vi "Create Installer.vi"(0 "Project Refnum":refnum<vi>, 5 "Build specification name":string, 11 "error in (no error)":errorcluster) -> (4 "Project Refnum Out":refnum<vi>, 15 "error out":errorcluster)   [LabVIEW 2021, in "G-Plugin Editor.lvlib"]
uses:
  G-Plugin Editor.lvlib
  <vilib>/AppBuilder/IB_Classes/Installer/Installer.lvclass
  <vilib>/AppBuilder/AB_API/common/AB_API Build Object Type.ctl
  <vilib>/AppBuilder/IB_Classes/Source/IB_Source.ctl
  <vilib>/AppBuilder/IB_Classes/Source/Container/Build/PackedLib/IB_PackedLib.lvclass
  C:/Program Files/National Instruments/LabVIEW 2021/vi.lib/AppBuilder/IB_Classes/Source/IB_Source.lvclass
  <vilib>/AppBuilder/IB_Classes/Destination/absFolder/absFolder.lvclass
  C:/Program Files/National Instruments/LabVIEW 2021/vi.lib/AppBuilder/IB_Classes/Destination/IB_Destination.lvclass
  <vilib>/AppBuilder/IB_Classes/Source/IB_Source.lvclass
  <vilib>/AppBuilder/IB_Classes/Destination/IB_Destination.lvclass
panel:
  out "Class out":refnum<class "Installer.lvclass">
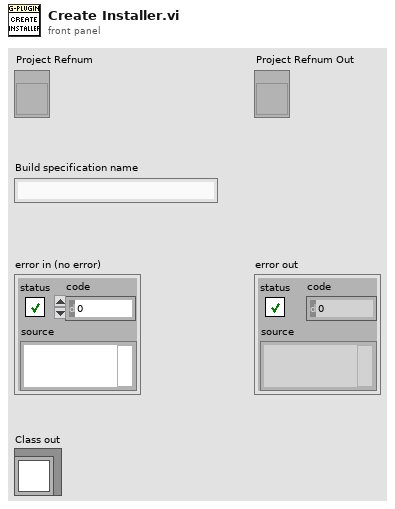
[diagram p1: front panel]
types:
  T1 = typedef "IB_Source.ctl" = cluster{"name":string, "sourceTag":string, "destTag":string, "path":path, "eng_installPath":string, "UI_inBuild?":bool, "str ref?":bool}
  T2 = typedef "AB_API Build Object Type.ctl" = enum16{"Source Distribution", "DLL", "EXE", "Installer", "Zip File", "RESTful WS", "RTEXE", "Packed Library", "C Generation ", ".NET Interop Assembly"}
  T3 = typedef "ItemRef.ctl" = u64
  T4 = typedef "IB_Installer.ctl" = cluster{"Destination":refnum<class "IB_Destination.lvclass">[], "Source":refnum<class "IB_Source.lvclass">[], "buildObject":T3, "defaultDir":string, "platform":string, "author":string, "productName":string, "buildSpecName":string, "hide":bool, "requireLVDevSys":bool, "autoIncrement":bool, "includeError":bool, "readmeID":string, "buildLocation":path, "readmePath":path, "mediaSize":u16, "language":T5, "productVersion":T6, "preview":bool, "programmatic":bool, "progressBarEvents":T7, "userLog_Path":path, "shortcutAddresses":T9[], "EXE_Install Address":string, "EXE_Uninstall Address":string, "additional NIPaths":refnum<class "Dest_NI_NIPath.lvclass">[], "web service itemIDs":string[], "installerName":string}
  T5 = typedef "CDK_sTypeDef_Languages.ctl" = u16
  T6 = typedef "CDK_sTypeDef_ProductVersion.ctl" = cluster{"Major":u8, "Minor":u8, "Update":u16}
  T7 = typedef "provcom_ProgressBar_Events.ctl" = cluster{"newJob":refnum<user-event>, "newItem":refnum<user-event>, "errorMsg":T8, "cancel":refnum<user-event>}
  T8 = typedef "mxLvBuildError.ctl" = refnum<user-event>
  T9 = typedef "CDK_sTypeDef_ShortcutAddress.ctl" = cluster{"file":string, "shortcut":string}
  T10 = typedef "IB_Destination.ctl" = cluster{"name":string, "unlock":bool, "parentTag":string, "destTag":string, "eng_installPath":string}
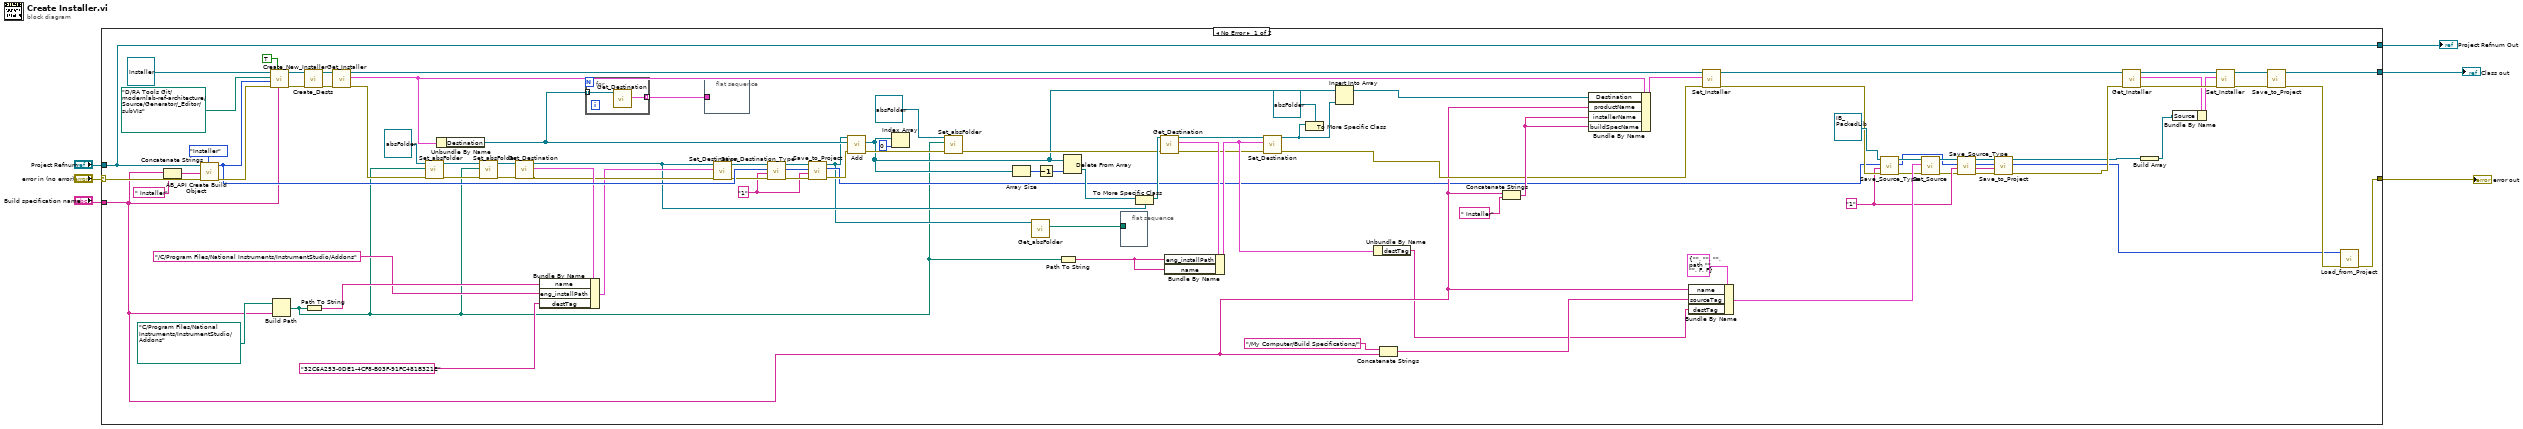
[diagram p0: block diagram]
diagram:
  n1 = case shown="No Error" "error in (no error)" {
    selector: "error in (no error)" -> [w100 w105]
    tunnel: [w72 w105] -> w6
    tunnel: "Build specification name" -> [w34 _]
    tunnel: "Project Refnum" -> [w91 w104]
    tunnel: [w88 _] -> w2
    tunnel: [w91 w104] -> w1
    frame No Error {
      w28 = "1" ("index in")
      w59 = "1" ("index")
      n2 = Concatenate Strings(w34, " Installer" ("string")) -> (w89:string)
      n3 = call <vilib>:"AB_API Create Build Object.vi"("Build object type"=AB_API_Build_Object_Type."Installer", "error in (no error)"=w100, "Build spec name"=w89, "Project Refnum"=w91) -> ("error out"=w97:errorcluster, "Build object"=w85:T3)  [unwired: 1 in, 5 out]
      n4 = call-dynamic "Create_New_Installer.vi"("buildSpecName"=w34, "Programmatic? (false)"=TRUE, "error in (no error)"=w97, "buildObject"=w85, "Destination Path"=path "D:/RA Tools Git/modernlab-ref-architecture/Source/Generator/_Editor/subVIs", "Class in"=refnum<class "Installer.lvclass"> refnum) -> ("error out"=w76:errorcluster, "Class out"=w93:refnum<class "Installer.lvclass">)  [unwired: 4 in]
      n5 = Build Path(base path=path "C:/Program Files/National Instruments/InstrumentStudio/Addons", name or relative path=w34) -> (appended path=w9:path)
      n6 = call-dynamic "Create_Dests.vi"("error in (no error)"=w76, "Class in"=w93) -> ("error out"=w81:errorcluster, "Class out"=w82:refnum<class "Installer.lvclass">)  [unwired: 8 in]
      n7 = Path To String(path=w9) -> (string=w44:string)
      n8 = call <vilib>:"Get_Installer.vi"("error in (no error)"=w81, "Installer in"=w82) -> ("error out"=w62:errorcluster, "data"=w71:T4, "Installer out"=w80:refnum<class "Installer.lvclass">)  [unwired: 7 in]
      n9 = call <vilib>:"Set_absFolder.vi"("error in (no error)"=w62, "Path"=w9, "absFolder in"=refnum<class "absFolder.lvclass"> refnum) -> ("error out"=w16:errorcluster, "absFolder out"=w19:refnum<class "absFolder.lvclass">)  [unwired: 7 in]
      n10 = Unbundle By Name(w71) -> ("Destination"=w61:refnum<class "IB_Destination.lvclass">[])
      n11 = call <vilib>:"Set_absFolder.vi"("error in (no error)"=w16, "Path"=w9, "absFolder in"=w19) -> ("error out"=w17:errorcluster, "absFolder out"=w18:refnum<class "absFolder.lvclass">)  [unwired: 7 in]
      n12 = call <vilib>:"Get_Destination.vi"("error in (no error)"=w17, "IB_Destination in"=w18) -> ("error out"=w78:errorcluster, "data"=w79:T10, "IB_Destination out"=w57:refnum<class "absFolder.lvclass">)  [unwired: 7 in]
      n13 = Bundle By Name(cluster=w79, "name"=w44, "eng_installPath"="/C/Program Files/National Instruments/InstrumentStudio/Addons", "destTag"="32C6A253-0DE1-4CF8-B03F-91FC481B321E" ("Build specification name")) -> (w77:T10)
      n14 = for {
        tunnel: w61 -> [w103] mode=indexing
        tunnel: [w102] -> w74 mode=indexing
        n15 = call <vilib>:"Get_Destination.vi"("IB_Destination in"=w103) -> ("data"=w102:T10)  [unwired: 8 in, 2 out]
      }
      n16 = flat-sequence {
        tunnel: w74 -> [_]
        frame #0 {
        }
      }
      n17 = call <vilib>:"Set_Destination.vi"("error in (no error)"=w78, "data"=w77, "IB_Destination in"=w57) -> ("error out"=w84:errorcluster, "IB_Destination out"=w87:refnum<class "absFolder.lvclass">)  [unwired: 7 in]
      n18 = call-dynamic "Save_Destination_Type.vi"("error in (no error)"=w84, "index"=w59, "buildObject"=w85, "absFolder in"=w87) -> ("error out"=w83:errorcluster, "buildObject out"=w65:T3, "absFolder out"=w86:refnum<class "absFolder.lvclass">)  [unwired: 4 in, 1 out]
      n19 = call-dynamic "Save_to_Project.vi"("error in (no error)"=w83, "index"=w59, "buildObject"=w65, "absFolder in"=w86) -> ("error out"=w60:errorcluster, "buildObject out"=w15:T3, "absFolder out"=w14:refnum<class "absFolder.lvclass">)  [unwired: 3 in, 2 out]
      n20 = call-dynamic "Add.vi"("error in (no error)"=w60, "Destinations in"=w61, "absFolder in"=w14) -> ("error out"=w48:errorcluster, "Destinations out"=w12:refnum<class "IB_Destination.lvclass">[])  [unwired: 5 in, 2 out]
      n21 = Index Array(array=w12, index=0) -> ()  [unwired: 1 out]
      n22 = call <vilib>:"Set_absFolder.vi"("Path"=w9, "absFolder in"=refnum<class "absFolder.lvclass"> refnum) -> ()  [unwired: 8 in, 2 out]
      n23 = Array Size(array=w12) -> (size(s)=w55:i32)
      n24 = call <vilib>:"Get_absFolder.vi"("absFolder in"=w14) -> ("Path"=w13:path)  [unwired: 8 in, 2 out]
      n25 = Decrement(x=w55) -> (x-1=w54:i32)
      n26 = Path To String(path=w9) -> (string=w50:string)
      n27 = Delete From Array(array=w12, index=w54) -> (deleted portion=w58:refnum<class "IB_Destination.lvclass">)  [unwired: 1 in, 1 out]
      n28 = flat-sequence {
        tunnel: w13 -> [_]
        frame #0 {
        }
      }
      n29 = To More Specific Class(target class=w57, reference=w58) -> (specific class reference=w53:refnum<class "absFolder.lvclass">)  [unwired: 1 in, 1 out]
      n30 = call <vilib>:"Get_Destination.vi"("error in (no error)"=w48, "IB_Destination in"=w53) -> ("error out"=w47:errorcluster, "data"=w51:T10, "IB_Destination out"=w52:refnum<class "absFolder.lvclass">)  [unwired: 7 in]
      n31 = Bundle By Name(cluster=w51, "eng_installPath"=w50, "name"=w50) -> (w49:T10)
      n32 = call <vilib>:"Set_Destination.vi"("error in (no error)"=w47, "data"=w49, "IB_Destination in"=w52) -> ("error out"=w46:errorcluster, "IB_Destination out"=w8:refnum<class "absFolder.lvclass">)  [unwired: 7 in]
      n33 = To More Specific Class(target class=refnum<class "absFolder.lvclass"> refnum ("absFolder in"), reference=w8) -> ()  [unwired: 1 in, 2 out]
      n34 = Insert Into Array(array=w12, new element=w8) -> (w56:refnum<class "IB_Destination.lvclass">[])  [unwired: 1 in]
      n35 = Unbundle By Name(w49) -> ("destTag"=w20:string)
      n36 = Concatenate Strings("/My Computer/Build Specifications/" ("Build specification name"), w34) -> (w33:string)
      n37 = Concatenate Strings(w34, " Installer" ("string")) -> (w70:string)
      n38 = Bundle By Name(cluster=w71, "Destination"=w56, "productName"=w34, "installerName"=w70, "buildSpecName"=w70) -> (w94:T4)
      n39 = Bundle By Name(cluster=T1 {"name"="", "sourceTag"="", "destTag"="", "path"=path "", "eng_installPath"="", "UI_inBuild?"=FALSE, "str ref?"=FALSE} ("data"), "name"=w34, "sourceTag"=w33, "destTag"=w20) -> (w67:T1)
      n40 = call <vilib>:"Set_Installer.vi"("error in (no error)"=w46, "data"=w94, "Installer in"=w80) -> ("error out"=w64:errorcluster, "Installer out"=w42:refnum<class "Installer.lvclass">)  [unwired: 7 in]
      n41 = call-dynamic "Save_Source_Type.vi"("error in (no error)"=w64, "index in"=w28, "buildObject"=w15, "Class in"=refnum<class "IB_PackedLib.lvclass"> refnum) -> ("error out"=w66:errorcluster, "buildObject out"=w23:T3, "Class out"=w68:refnum<class "IB_PackedLib.lvclass">)  [unwired: 4 in, 1 out]
      n42 = call <vilib>:"Set_Source.vi"("error in (no error)"=w66, "data"=w67, "IB_Source in"=w68) -> ("error out"=w27:errorcluster, "IB_Source out"=w30:refnum<class "IB_PackedLib.lvclass">)  [unwired: 7 in]
      n43 = call-dynamic "Save_Source_Type.vi"("error in (no error)"=w27, "index in"=w28, "buildObject"=w23, "Class in"=w30) -> ("error out"=w26:errorcluster, "index out"=w25:string, "buildObject out"=w24:T3, "Class out"=w29:refnum<class "IB_PackedLib.lvclass">)  [unwired: 4 in]
      n44 = call-dynamic "Save_to_Project.vi"("error in (no error)"=w26, "index in"=w25, "buildObject"=w24, "Class in"=w29) -> ("error out"=w31:errorcluster, "buildObject out"=w22:T3, "Class out"=w21:refnum<class "IB_PackedLib.lvclass">)  [unwired: 3 in, 2 out]
      n45 = call <vilib>:"Get_Installer.vi"("error in (no error)"=w31, "Installer in"=w42) -> ("error out"=w39:errorcluster, "data"=w37:T4, "Installer out"=w41:refnum<class "Installer.lvclass">)  [unwired: 7 in]
      n46 = Build Array(w21) -> (w35:refnum<class "IB_PackedLib.lvclass">[])
      n47 = Bundle By Name(cluster=w37, "Source"=w35) -> (w36:T4)
      n48 = call <vilib>:"Set_Installer.vi"("error in (no error)"=w39, "data"=w36, "Installer in"=w41) -> ("error out"=w38:errorcluster, "Installer out"=w40:refnum<class "Installer.lvclass">)  [unwired: 7 in]
      n49 = call-dynamic "Save_to_Project.vi"("error in (no error)"=w38, "Installer in"=w40) -> ("error out"=w73:errorcluster, "Installer out"=w88:refnum<class "Installer.lvclass">)  [unwired: 8 in]
      n50 = call <vilib>:"Load_from_Project.vi"("error in (no error)"=w73, "Object"=w22) -> ("error out"=w72:errorcluster)  [unwired: 8 in, 1 out]
    }
    frame Error {
    }
  }
  "error out" <- w6
  "Project Refnum Out" <- w1
  "Class out" <- w2
